vi "Experiment header-Save_Load config file data.vi"(5 "Header file actions":T1=enum."Write All", 7 "Header file sections":T22=enum."LOGIN", 8 "error in (no error)":errorcluster, 9 "All header parameters in":T2 {"VOLUME IMAGING"."Plane Mode" items=["XY Plane", "XZ Plane", "YZ Plane", "arbitraryplane"]; "VOLUME IMAGING"."Basic Image meta data"."Frame Size" items=["100X100"=100, "128X128"=128, "200X200"=200, "256X256"=256, "512X512"=512, "1024x1024"=1024, "2048x2048"=2048]; "AOL Z-STACK"."Hdr Basic Image meta data"."Frame Size" items=["100X100"=100, "128X128"=128, "200X200"=200, "256X256"=256, "512X512"=512, "1024x1024"=1024, "2048x2048"=2048]; "MOTOR Z-STACK"."Hdr Basic Image meta data"."Frame Size" items=["100X100"=100, "128X128"=128, "200X200"=200, "256X256"=256, "512X512"=512, "1024x1024"=1024, "2048x2048"=2048]; "FUNCTIONAL IMAGING"."Plane Mode" items=["XY Plane", "XZ Plane", "YZ Plane", "arbitraryplane"]; "FUNCTIONAL IMAGING"."Basic Image meta data"."Frame Size" items=["100X100"=100, "128X128"=128, "200X200"=200, "256X256"=256, "512X512"=512, "1024x1024"=1024, "2048x2048"=2048]; "TIME SERIES"."Basic Image meta data"."Frame Size" items=["100X100"=100, "128X128"=128, "200X200"=200, "256X256"=256, "512X512"=512, "1024x1024"=1024, "2048x2048"=2048]}, 11 "Experiment data folder path":path) -> (0 "error out":errorcluster, 1 "All header parameters out":T2 {"VOLUME IMAGING"."Plane Mode" items=["XY Plane", "XZ Plane", "YZ Plane", "arbitraryplane"]; "VOLUME IMAGING"."Basic Image meta data"."Frame Size" items=["100X100"=100, "128X128"=128, "200X200"=200, "256X256"=256, "512X512"=512, "1024x1024"=1024, "2048x2048"=2048]; "AOL Z-STACK"."Hdr Basic Image meta data"."Frame Size" items=["100X100"=100, "128X128"=128, "200X200"=200, "256X256"=256, "512X512"=512, "1024x1024"=1024, "2048x2048"=2048]; "MOTOR Z-STACK"."Hdr Basic Image meta data"."Frame Size" items=["100X100"=100, "128X128"=128, "200X200"=200, "256X256"=256, "512X512"=512, "1024x1024"=1024, "2048x2048"=2048]; "FUNCTIONAL IMAGING"."Plane Mode" items=["XY Plane", "XZ Plane", "YZ Plane", "arbitraryplane"]; "FUNCTIONAL IMAGING"."Basic Image meta data"."Frame Size" items=["100X100"=100, "128X128"=128, "200X200"=200, "256X256"=256, "512X512"=512, "1024x1024"=1024, "2048x2048"=2048]; "TIME SERIES"."Basic Image meta data"."Frame Size" items=["100X100"=100, "128X128"=128, "200X200"=200, "256X256"=256, "512X512"=512, "1024x1024"=1024, "2048x2048"=2048]})   [LabVIEW 2020]
doc: "This self-contained module handles all header files save/write operations.\nIt can generate a number of different header files containing different parameters.\nEach different type of header file has its own type defined cluster of parameters.\nThe functionality is fully self-scalable such as when new parameters are added or parameters are deleted or renamed in the typedef clusters this is all handled automatically without the need for further updates to this module."
uses:
  <vilib>/Utility/config.llb/NI_LVConfig.lvlib
  <vilib>/Utility/config.llb/Write Key (Double).vi
  Typedefs/Header file type enum.ctl
  Typedefs/Header subclusters/Header params -Login.ctl
  Misc/Experiment Type.ctl
  Typedefs/Header subclusters/Header params-Global Parameters.ctl
  Typedefs/Header subclusters/Header params-Imaging Modes.ctl
  Typedefs/Header subclusters/Header params-Basic image meta data.ctl
  Typedefs/Header subclusters/Header params-Time Series.ctl
  Typedefs/Header subclusters/Header params-Functional Imaging.ctl
  Typedefs/Reference source.ctl
  Typedefs/Header subclusters/Header params-Movement correction.ctl
  Typedefs/Header subclusters/Header params-Calibration Setup.ctl
  Typedefs/Header subclusters/Header params-statistics.ctl
  Misc/Biology Information.ctl
  Typedefs/Header subclusters/Header params-Motor Z-stack.ctl
  Typedefs/Header subclusters/Header params-AOL Z-stack.ctl
  Typedefs/Header parameters cluster-ALL.ctl
  Typedefs/Header file actions.ctl
  <vilib>/Utility/config.llb/Read Key (Double).vi
  Typedefs/Functional Mode.ctl
  Typedefs/AOL modes.ctl
  Typedefs/Plane Mode.ctl
  Typedefs/Frame Size.ctl
  Typedefs/Header subclusters/Header params-calibration data.ctl
  Typedefs/Header file sections.ctl
panel:
  out "error":errorcluster
  # "Actual FOV ------>\n(not norm FOFV)"
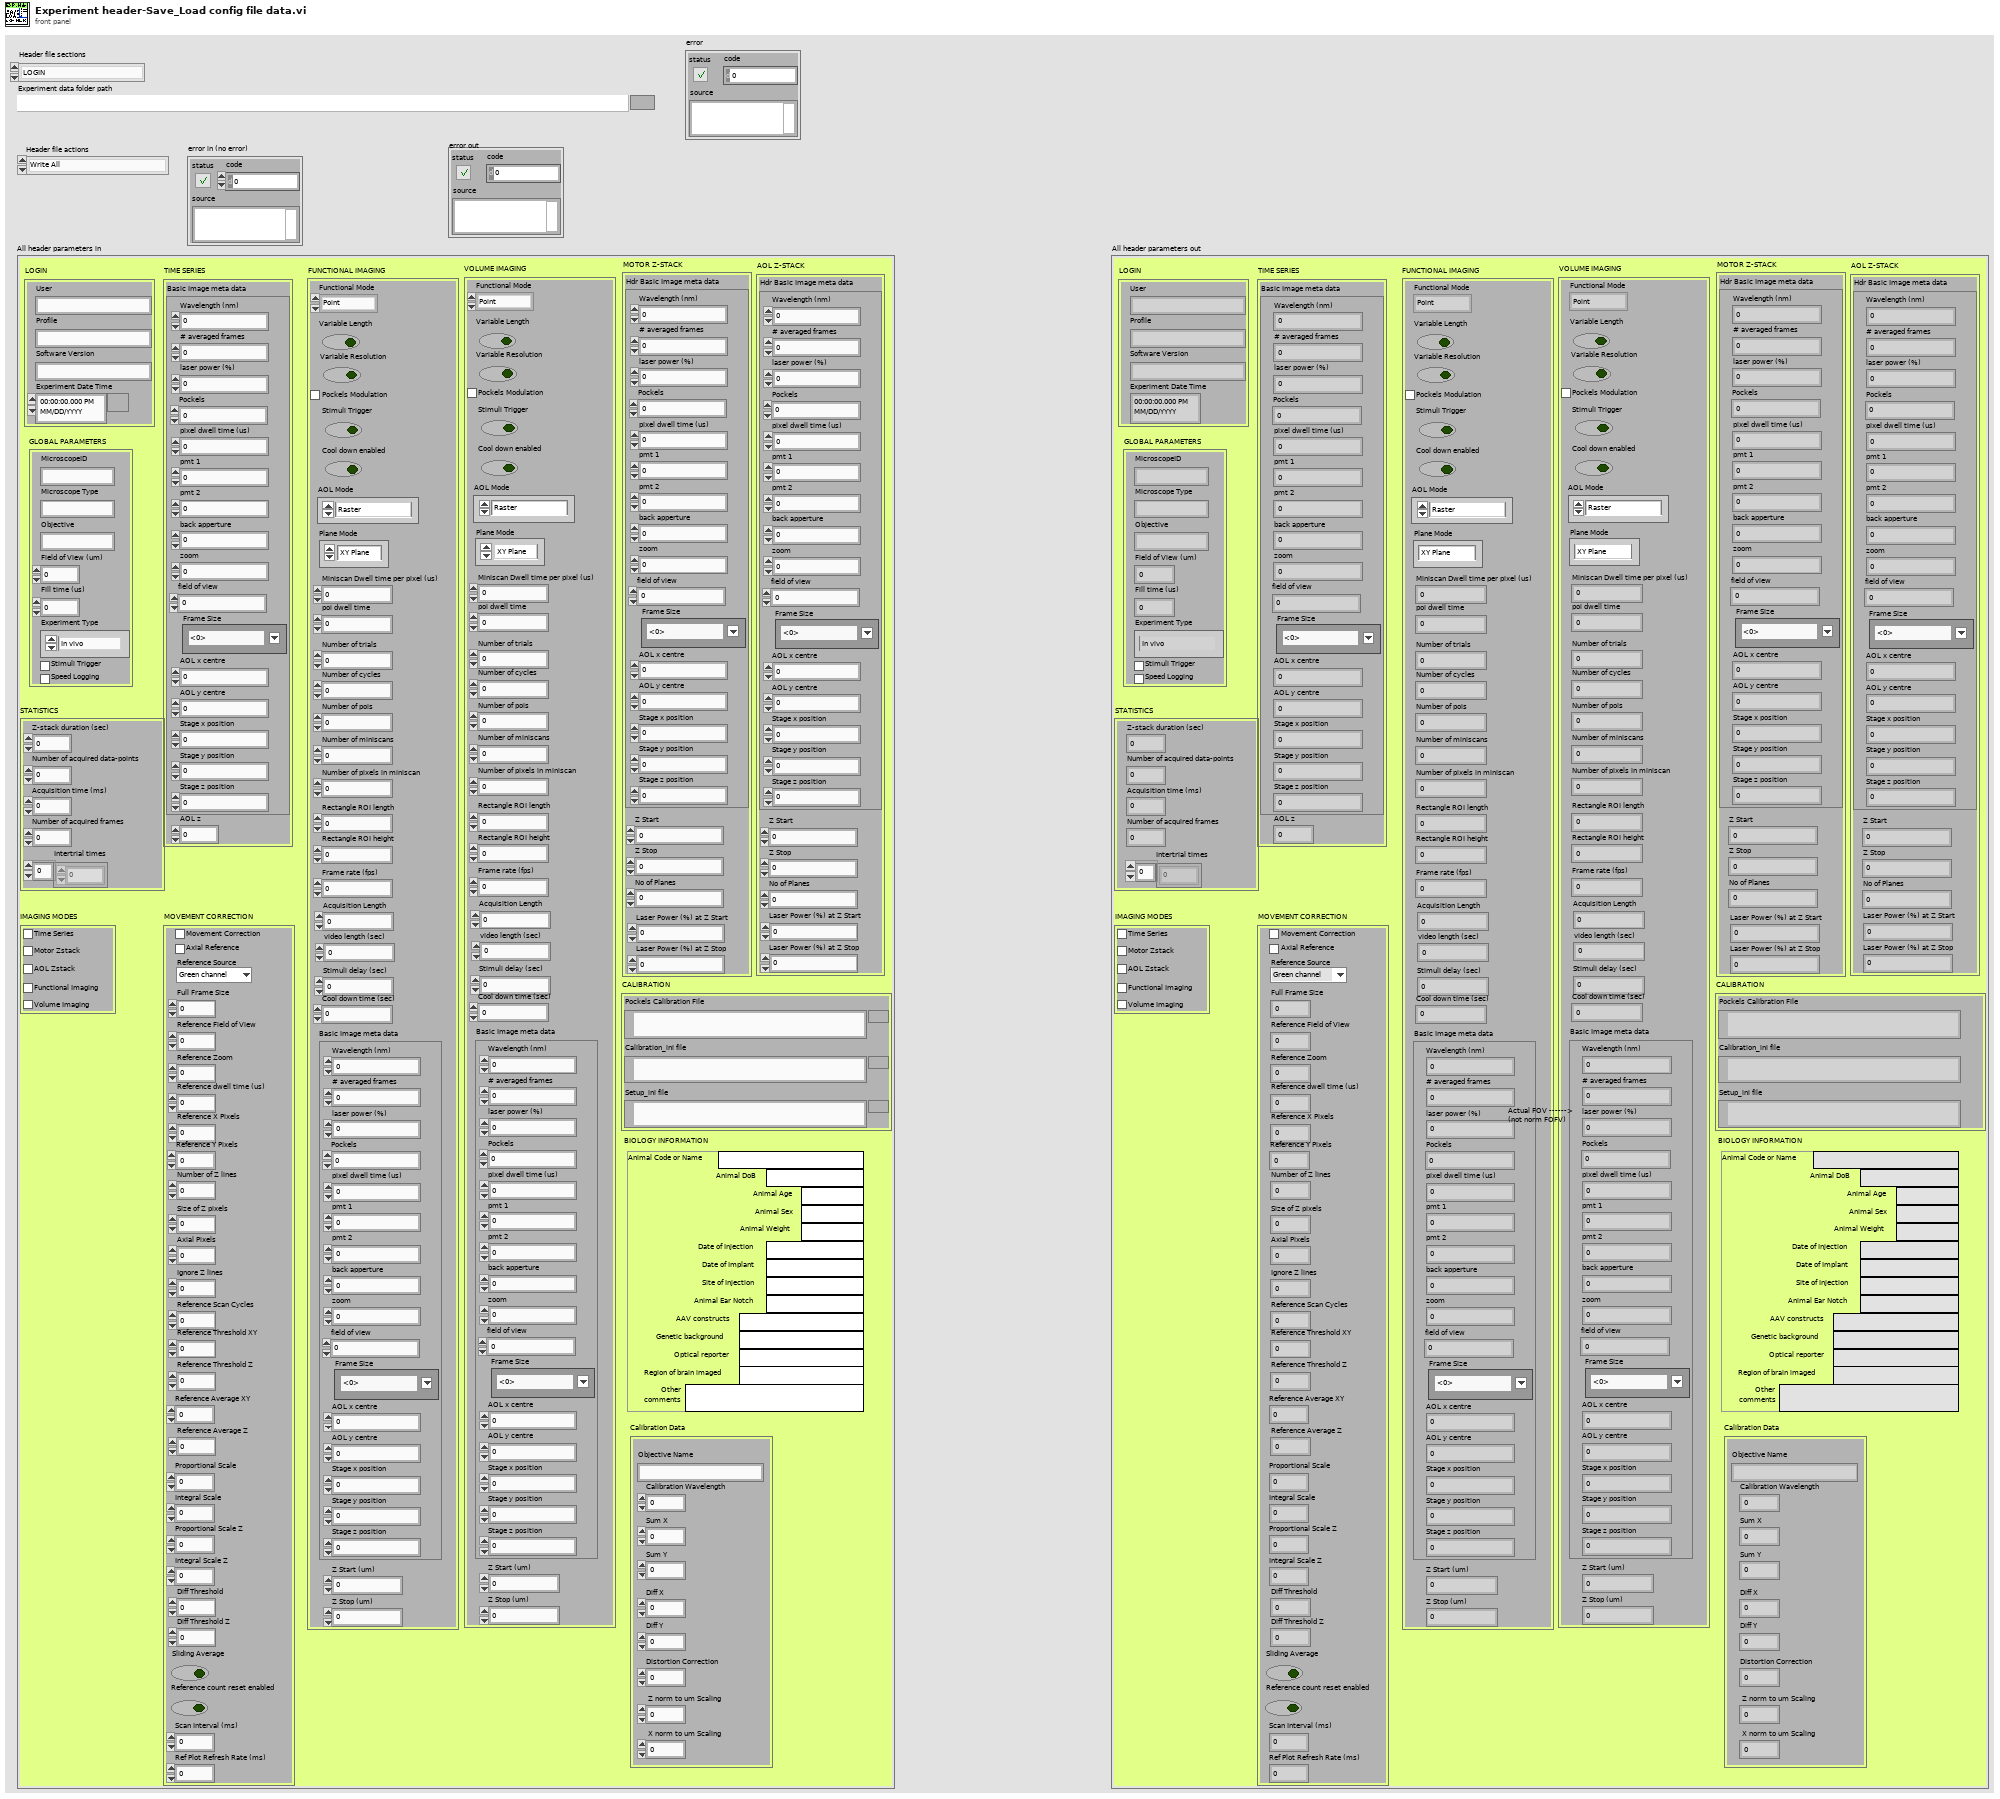
[diagram p1: front panel]
types:
  T1 = typedef "Header file actions.ctl" = enum16{"Create", "Open", "Read All", "Read Section", "Write All", "Write Section", "Close"}
  T2 = typedef "Header parameters cluster-ALL.ctl" = cluster{"LOGIN":T3, "GLOBAL PARAMETERS":T4, "IMAGING MODES":T6, "TIME SERIES":T7, "MOTOR Z-STACK ":T10, "AOL Z-STACK":T11, "FUNCTIONAL IMAGING":T12, "VOLUME IMAGING":T12, "MOVEMENT CORRECTION":T16, "CALIBRATION":T18, "STATISTICS":T19, "BIOLOGY INFORMATION":T20, "Calibration Data":T21}
  T3 = typedef "Header params -Login.ctl" = cluster{"User":string, "Profile":string, "Software Version":string, "Experiment Date Time":timestamp}
  T4 = typedef "Header params-Global Parameters.ctl" = cluster{"MicroscopeID":string, "Microscope Type":string, "Objective":string, "Field of View (um)":dbl, "Fill time (us)":dbl, "Experiment Type":T5, "Stimuli Trigger":bool, "Speed Logging":bool}
  T5 = typedef "Experiment Type.ctl" = enum16{"In vivo", "In vitro", "Testing", "Calibration", "Other"}
  T6 = typedef "Header params-Imaging Modes.ctl" = cluster{"Time Series":bool, "Motor Zstack":bool, "AOL Zstack":bool, "Functional Imaging":bool, "Volume Imaging":bool}
  T7 = typedef "Header params-Time Series.ctl" = cluster{"Basic Image meta data":T8, "AOL z":dbl}
  T8 = typedef "Header params-Basic image meta data.ctl" = cluster{"Wavelength (nm)":dbl, "# averaged frames":dbl, "laser power (%)":dbl, "Pockels":dbl, "pixel dwell time (us)":dbl, "pmt 1":dbl, "pmt 2":dbl, "back apperture":dbl, "zoom":dbl, "field of view":dbl, "Frame Size":T9, "AOL x centre":dbl, "AOL y centre":dbl, "Stage x position":dbl, "Stage y position":dbl, "Stage z position":dbl}
  T9 = typedef "Frame Size.ctl" = u16
  T10 = typedef "Header params-Motor Z-stack.ctl" = cluster{"Hdr Basic Image meta data":T8, "Z Start":dbl, "Z Stop":dbl, "No of Planes":i32, "Laser Power (%) at Z Start":dbl, "Laser Power (%) at Z Stop":dbl}
  T11 = typedef "Header params-AOL Z-stack.ctl" = cluster{"Hdr Basic Image meta data":T8, "Z Start":dbl, "Z Stop":dbl, "No of Planes":i32, "Laser Power (%) at Z Start":dbl, "Laser Power (%) at Z Stop":dbl}
  T12 = typedef "Header params-Functional Imaging.ctl" = cluster{"Functional Mode":T13, "Variable Length":bool, "Variable Resolution":bool, "Pockels Modulation":bool, "Stimuli Trigger":bool, "Cool down enabled":bool, "AOL Mode":T14, "Plane Mode":T15, "Miniscan Dwell time per pixel (us)":dbl, "poi dwell time":dbl, "Number of trials":dbl, "Number of cycles":dbl, "Number of pois":dbl, "Number of miniscans":dbl, "Number of pixels in miniscan":dbl, "Rectangle ROI length":dbl, "Rectangle ROI height":dbl, "Frame rate (fps)":dbl, "Acquisition Length":dbl, "video length (sec)":dbl, "Stimuli delay (sec)":dbl, "Cool down time (sec)":dbl, "Basic Image meta data":T8, "Z Start (um)":dbl, "Z Stop (um)":dbl}
  T13 = typedef "Functional Mode.ctl" = enum16{"Point", "Line", "Patch", "Plane", "Volume"}
  T14 = typedef "AOL modes.ctl" = enum16{"Raster", "Structural", "Pointing", "Mini Scan", "Alignment"}
  T15 = typedef "Plane Mode.ctl" = u16
  T16 = typedef "Header params-Movement correction.ctl" = cluster{"Movement Correction":bool, "Axial Reference":bool, "Reference Source":T17, "Full Frame Size":dbl, "Reference Field of View":dbl, "Reference Zoom":dbl, "Reference dwell time (us)":dbl, "Reference X Pixels":dbl, "Reference Y Pixels":dbl, "Number of Z lines":dbl, "Size of Z pixels":dbl, "Axial Pixels":dbl, "Ignore Z lines":dbl, "Reference Scan Cycles":dbl, "Reference Threshold XY":dbl, "Reference Threshold Z":dbl, "Reference Average XY":dbl, "Reference Average Z":dbl, "Proportional Scale":dbl, "Integral Scale":dbl, "Proportional Scale Z":dbl, "Integral Scale Z":dbl, "Diff Threshold":dbl, "Diff Threshold Z":dbl, "Sliding Average":bool, "Reference count reset enabled":bool, "Scan Interval (ms)":dbl, "Ref Plot Refresh Rate (ms)":dbl}
  T17 = typedef "Reference source.ctl" = enum16{"Green channel", "Red channel"}
  T18 = typedef "Header params-Calibration Setup.ctl" = cluster{"Pockels Calibration File":path, "Calibration_ini file":path, "Setup_ini file":path}
  T19 = typedef "Header params-statistics.ctl" = cluster{"Z-stack duration (sec)":dbl, "Number of acquired data-points":dbl, "Acquisition time (ms)":dbl, "Number of acquired frames":dbl, "Intertrial times":dbl[]}
  T20 = typedef "Biology Information.ctl" = cluster{"Animal Code or Name":string, "Animal DoB":string, "Animal Age":string, "Animal Sex":string, "Animal Weight":string, "Date of Injection":string, "Date of Implant":string, "Site of Injection":string, "Animal Ear Notch":string, "AAV constructs":string, "Genetic background":string, "Optical reporter":string, "Region of brain imaged":string, "Other \ncomments":string}
  T21 = typedef "Header params-calibration data.ctl" = cluster{"Objective Name":string, "Calibration Wavelength":dbl, "Sum X":dbl, "Sum Y":dbl, "Diff X":dbl, "Diff Y":dbl, "Distortion Correction":dbl, " Z norm to um Scaling":dbl, " X norm to um Scaling":dbl}
  T22 = typedef "Header file sections.ctl" = enum16{"ALL SECTIONS", "LOGIN", "GLOBAL PARAMETERS", "CALIBRATION DATA", "IMAGING MODES", "TIME SERIES", "MOTOR Z-STACK", "AOL Z-STACK", "FUNCTIONAL IMAGING", "VOLUME IMAGING", "ARBOREAL SCANNING", "MULTIBEAM PARAMETERS", "MOVEMENT CORRECTION", "CALIBRATION", "STATISTICS", "BIOLOGY INFORMATION", "PARAMETER SWEEP"}
  T23 = typedef "Header file section refs.ctl" = cluster{"Section Name":string, "Section Ref":refnum<vi>, "Section Controls[]":refnum<vi>[]}
  T24 = typedef "Fixed strings.ctl" = cluster{"ROI file name":string, "Normalised ROI file name":string, "Zplane Pockels values file name":string, "Functional data folder name":string, "Experiment Header file name":string, "Z-stack images folder name":string, "Groups setup rel. path":string, "Groups text file rel. path":string, "TDMS files folder name (F.img)":string, "TDMS files folder name (V.acq)":string, "TDMS files folder name (Pl.acq)":string, "Cycle rel times sequence file":string, "Dynamically called VIs folder name":string, "Time Series folder base name":string, "Parameter Sweep":string}
  T25 = typedef "Header parameters cluster-ALL.ctl" = cluster{"LOGIN":T3, "GLOBAL PARAMETERS":T4, "IMAGING MODES":T6, "TIME SERIES":T7, "MOTOR Z-STACK ":T10, "AOL Z-STACK":T11, "FUNCTIONAL IMAGING":T12, "VOLUME IMAGING":T12, "MOVEMENT CORRECTION":T16, "CALIBRATION":T18, "STATISTICS":T19, "BIOLOGY INFORMATION":T20, "Calibration Data":T21, "Parameter Sweep Settings":T26}
  T26 = typedef "Header params-Parameter Sweep.ctl" = cluster{"Parameter Sweep Steps":T27, "Parameter Sweep":T28, "# Sw. Planes":i32, "Basic image meta-data":T8}
  T27 = typedef "Parameter Sweep Steps.ctl" = cluster{"MB Sep Start":dbl, "MB Sep Stop":dbl, "MB Sep Step":dbl}
  T28 = typedef "Parameter sweep modes.ctl" = enum16{"None Selected", "Dwell Time [us]"}
  T29 = typedef "Header file type enum.ctl" = enum16{"All parameters", "Login", "Global Parameters", "Imaging Modes", "Time Series", "Motor Zstack", "AOL Zstack", "Functional Imaging", "Movement Correction", "Calibration Setup", "Statistics", "Biology Information"}
  T30 = typedef "NI_LVConfig.lvlib/Config Data RefNum.ctl" = refnum<k1>
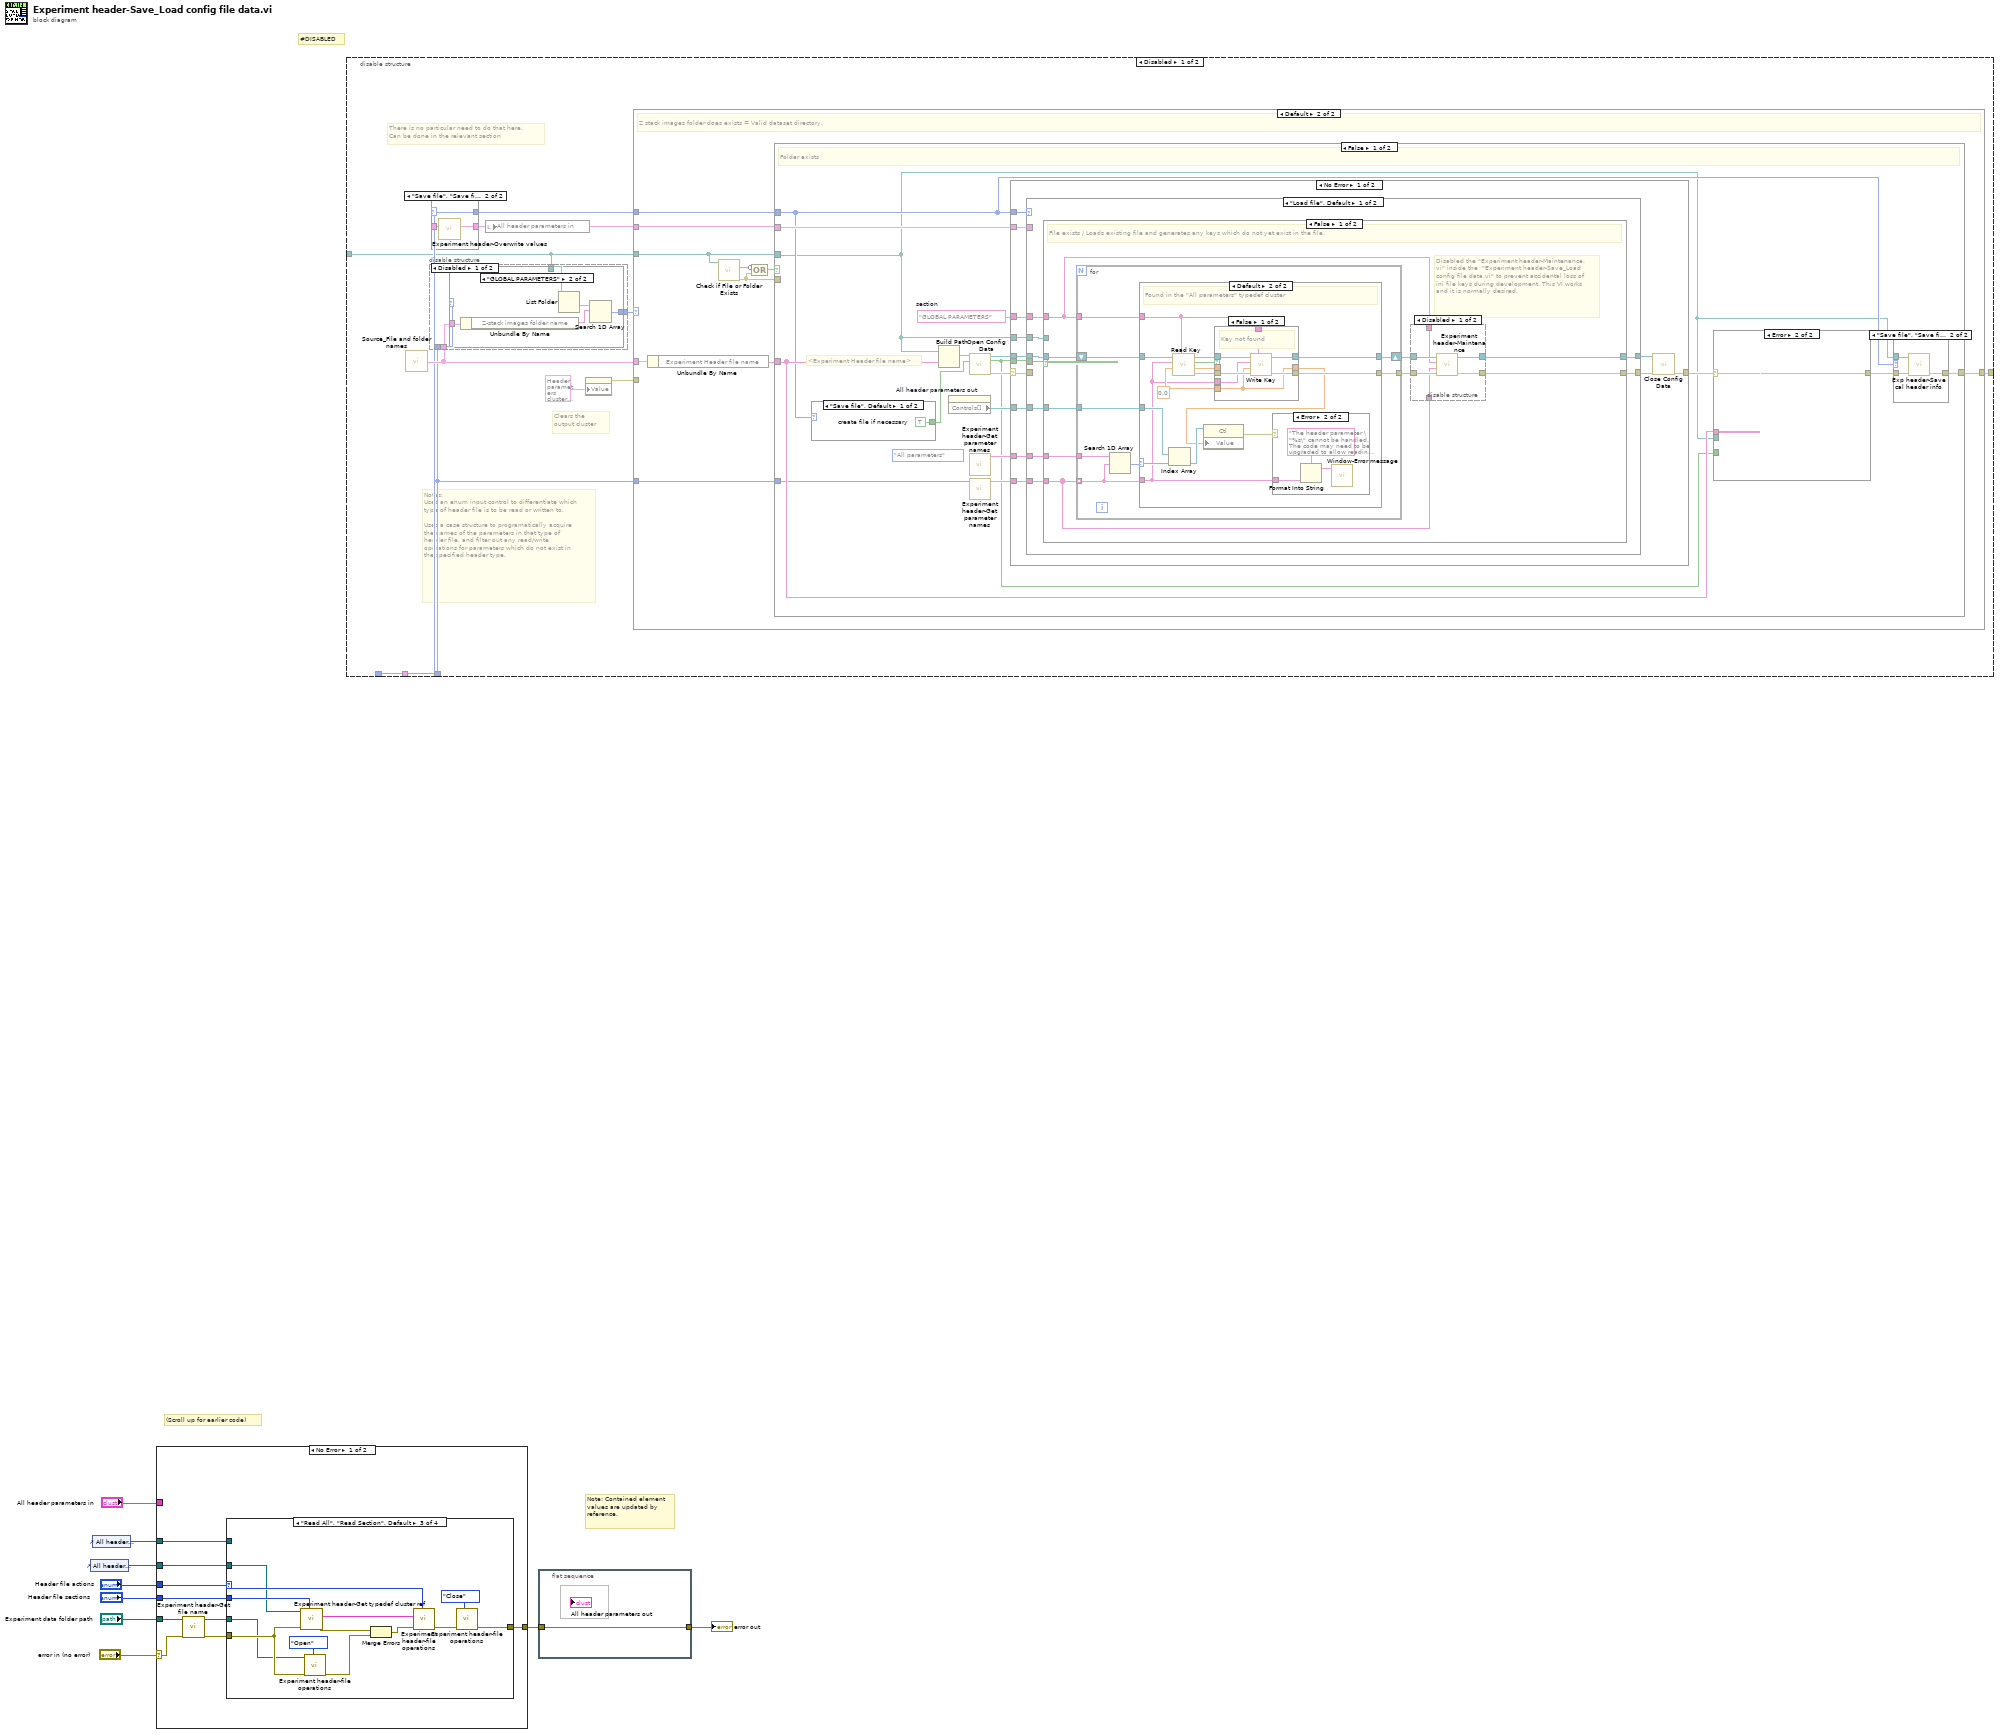
[diagram p0: block diagram]
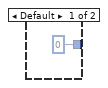
[diagram p3: hidden frame]
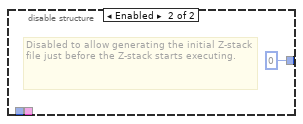
[diagram p4: hidden frame]
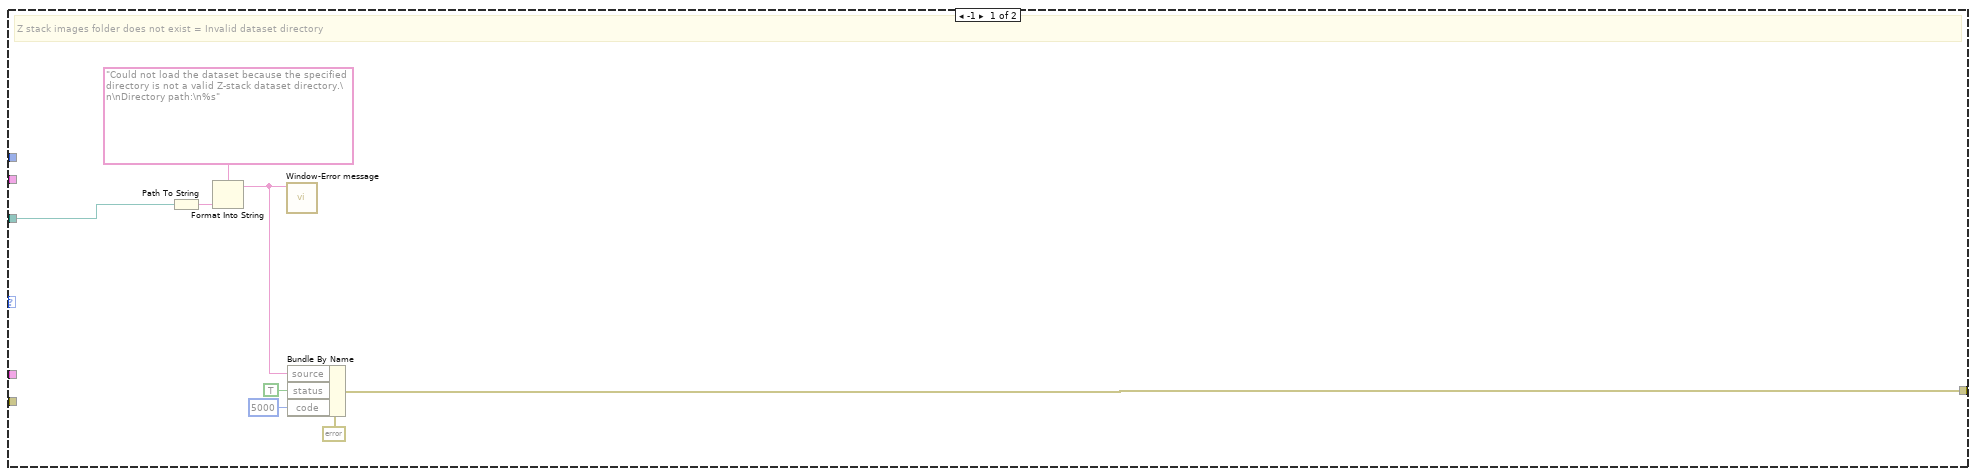
[diagram p5: hidden frame]
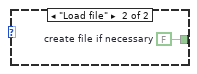
[diagram p7: hidden frame]
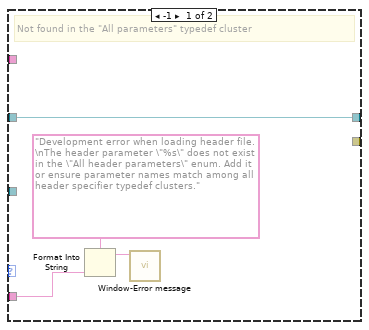
[diagram p9: hidden frame]
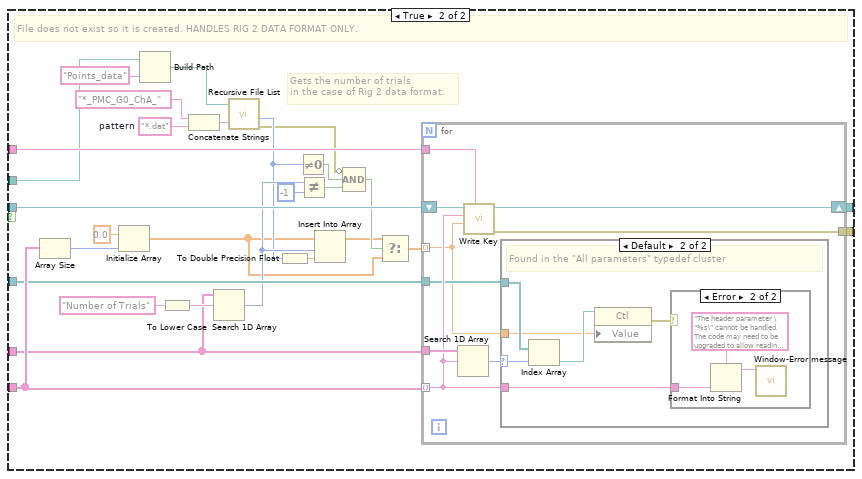
[diagram p12: hidden frame]
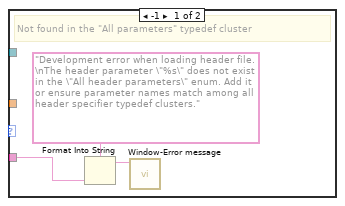
[diagram p13: hidden frame]
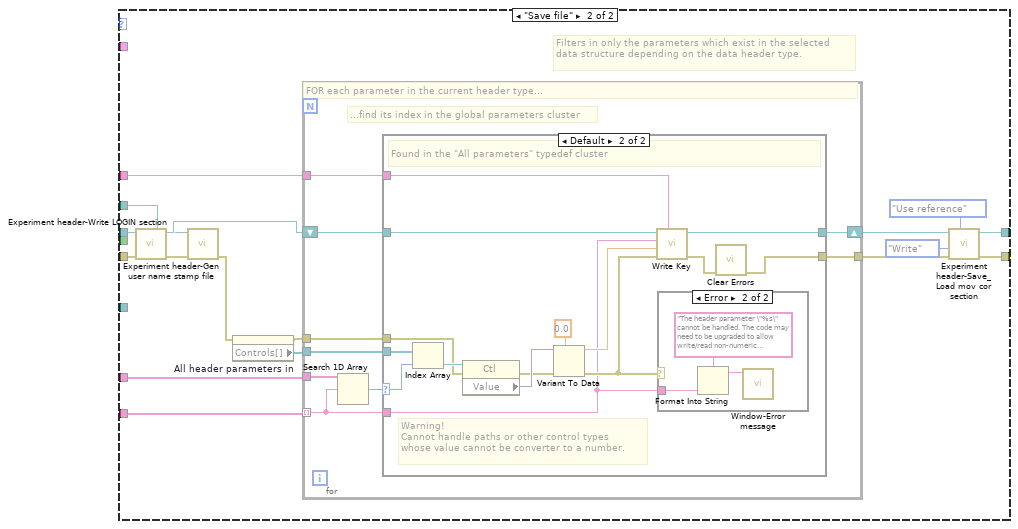
[diagram p15: hidden frame]
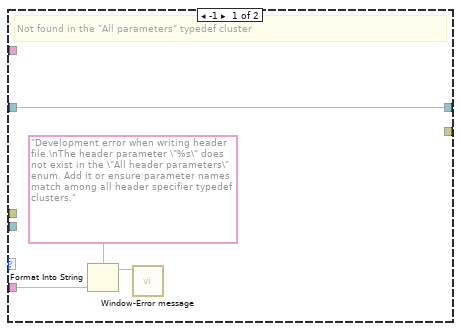
[diagram p16: hidden frame]
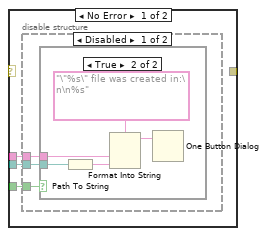
[diagram p19: hidden frame]
diagram:
  # "Note: Contained element values are updated by reference."
  # "(Scroll up for earlier code)"
  # "#DISABLED"
  n1 = control-ref of="All header parameters out"() -> (w3:refnum<vi>)
  n2 = control-ref of="All header parameters in"() -> (w4:refnum<vi>)
  n3 = case shown="No Error" "error in (no error)" {
    selector: "error in (no error)" -> [w11 w53]
    tunnel: [w10 w53] -> w2
    tunnel: "Header file sections" -> [w15 _]
    tunnel: "All header parameters in" -> [_ _]
    tunnel: "Experiment data folder path" -> [w18 _]
    tunnel: "Header file actions" -> [w14 _]
    tunnel: w4 -> [w13 _]
    tunnel: w3 -> [w12 _]
    frame No Error {
      n4 = call "Experiment header-Get file name.vi"("error in (no error)"=w11, "Experiment data folder path"=w18) -> ("error out"=w17:errorcluster, "Header File Path"=w16:path)  [unwired: 8 in]
      n5 = case shown="\"Read All\", \"Read Section\", Default" w14 {
        selector: w14 -> [w21 w34 w48 _]
        tunnel: w17 -> [w22 w27 w45 w52]
        tunnel: w16 -> [w20 w33 w38 _]
        tunnel: w15 -> [_ w35 w47 _]
        tunnel: w13 -> [_ w23 _ _]
        tunnel: w12 -> [_ _ w37 _]
        tunnel: [w19 w24 w40 w50] -> w10
        frame "Create" {
          n6 = call "Experiment header-file operations.vi"("Header file actions"=w21, "error in (no error)"=w22, "Path"=w20) -> ("error out"=w19:errorcluster)  [unwired: 8 in]
        }
        frame "Write All", "Write Section" {
          n7 = call "Experiment header-Gen user name stamp file.vi"("error in (no error)"=w27, "Experiment data folder path"=w33) -> ("error out"=→"error":errorcluster)  [unwired: 9 in]
          n8 = call "Experiment header-Get typedef cluster ref.vi"("Header file sections"=w35, "All header parameters / Header module interface cluster"=w23) -> ("error out"=w31:errorcluster, "Section Refs"=w36:T23[])  [unwired: 6 in, 2 out]
          n9 = call "Experiment header-file operations.vi"("Header file actions"=Header_file_actions."Open", "error in (no error)"=w27, "Path"=w33) -> ("error out"=w30:errorcluster)  [unwired: 8 in]
          n10 = Merge Errors(w31, w30) -> (w29:errorcluster)
          n11 = call "Experiment header-file operations.vi"("Header file actions"=w34, "error in (no error)"=w29, "Section Refs"=w36) -> ("error out"=w25:errorcluster)  [unwired: 8 in]
          n12 = call "Experiment header-file operations.vi"("Header file actions"=Header_file_actions."Close", "error in (no error)"=w25) -> ("error out"=w24:errorcluster)  [unwired: 9 in]
        }
        frame "Read All", "Read Section", Default {
          n13 = call "Experiment header-Get typedef cluster ref.vi"("Header file sections"=w47, "error in (no error)"=w45, "All header parameters / Header module interface cluster"=w37) -> ("error out"=w44:errorcluster, "Section Refs"=w49:T23[])  [unwired: 5 in, 2 out]
          n14 = call "Experiment header-file operations.vi"("Header file actions"=Header_file_actions."Open", "error in (no error)"=w45, "Path"=w38) -> ("error out"=w42:errorcluster)  [unwired: 8 in]
          n15 = Merge Errors(w44, w42) -> (w43:errorcluster)
          n16 = call "Experiment header-file operations.vi"("Header file actions"=w48, "error in (no error)"=w43, "Section Refs"=w49) -> ("error out"=w39:errorcluster)  [unwired: 8 in]
          n17 = call "Experiment header-file operations.vi"("Header file actions"=Header_file_actions."Close", "error in (no error)"=w39) -> ("error out"=w40:errorcluster)  [unwired: 9 in]
        }
        frame "Close" {
          n18 = call "Experiment header-file operations.vi"("Header file actions"=Header_file_actions."Close", "error in (no error)"=w52) -> ("error out"=w50:errorcluster)  [unwired: 9 in]
        }
      }
    }
    frame Error {
    }
  }
  n19 = disable-structure shown="Disabled" {
    disable-tunnel: [w64 _] -> _
    disable-tunnel: _ -> [w59 _]
    disable-tunnel: _ -> [w58 _]
    disable-tunnel: _ -> [w57 _]
    disable-tunnel: _ -> [w54 _]
    frame Disabled {
      # "There is no particular need to do that here.\nCan be done in the relevant section"
      # "Clears the output cluster"
      # "Notes:\nUses an enum input control to differentiate which type of header file is to be read or written to.\n\nUses a case structure to programatically acquire the names of the parameters in that type of header file, and filter out any read/write operations for parameters which do not exist in the specified header type."
      n20 = call "Source_File and folder names.vi"() -> ("Fixed strings"=w62:T24)  [unwired: 1 in]
      n21 = disable-structure shown="Disabled" {
        disable-tunnel: w57 -> [w73 _]
        disable-tunnel: [w72 0 ("index of element")] -> w63
        disable-tunnel: w62 -> [w71 _]
        disable-tunnel: w54 -> [w70 _]
        frame Disabled {
          n22 = case shown="\"GLOBAL PARAMETERS\"" w70 {
            tunnel: w73 -> [_ w78]
            tunnel: [0 ("index of element") w77] -> w72
            tunnel: w71 -> [_ w75]
            frame Default {
            }
            frame "GLOBAL PARAMETERS" {
              n23 = Unbundle By Name(w75) -> ("Z-stack images folder name"=w76:string)
              n24 = List Folder(path=w78) -> (folder names=w79:string[])  [unwired: 3 in, 3 out]
              n25 = Search 1D Array(1D array=w79, element=w76) -> (index of element=w77:i32)  [unwired: 1 in]
            }
          }
        }
        frame Enabled {
          # "Disabled to allow generating the initial Z-stack file just before the Z-stack starts executing."
        }
      }
      n26 = case shown="\"Save file\", \"Save file as\"" w59 {
        selector: w59 -> [w66 w68]
        tunnel: [w65 w69] -> w56
        tunnel: [w66 w68] -> w60
        tunnel: w58 -> [w65 w67]
        frame Default {
        }
        frame "Save file", "Save file as" {
          n27 = call "Experiment header-Overwrite values.vi"("All header parameters in"=w67) -> ("All header parameters (FOV converted to um)"=w69:T25)  [unwired: 9 in, 1 out]
        }
      }
      n28 = local write "All header parameters in"(w56) -> ()
      n29 = property on="All header parameters out" class="Clust (strict)"("Value"=T2 {"LOGIN"={"User"="", "Profile"="", "Software Version"="", "Experiment Date Time"=timestamp(0 s since 1904-01-01)}, "GLOBAL PARAMETERS"={"MicroscopeID"="", "Microscope Type"="", "Objective"="", "Field of View (um)"=0.0, "Fill time (us)"=0.0, "Experiment Type"=enum."In vivo", "Stimuli Trigger"=FALSE, "Speed Logging"=FALSE}, "IMAGING MODES"={"Time Series"=FALSE, "Motor Zstack"=FALSE, "AOL Zstack"=FALSE, "Functional Imaging"=FALSE, "Volume Imaging"=FALSE}, "TIME SERIES"={"Basic Image meta data"={"Wavelength (nm)"=0.0, "# averaged frames"=0.0, "laser power (%)"=0.0, "Pockels"=0.0, "pixel dwell time (us)"=0.0, "pmt 1"=0.0, "pmt 2"=0.0, "back apperture"=0.0, "zoom"=0.0, "field of view"=0.0, "Frame Size"=0, "AOL x centre"=0.0, "AOL y centre"=0.0, "Stage x position"=0.0, "Stage y position"=0.0, "Stage z position"=0.0}, "AOL z"=0.0}, "MOTOR Z-STACK "={"Hdr Basic Image meta data"={"Wavelength (nm)"=0.0, "# averaged frames"=0.0, "laser power (%)"=0.0, "Pockels"=0.0, "pixel dwell time (us)"=0.0, "pmt 1"=0.0, "pmt 2"=0.0, "back apperture"=0.0, "zoom"=0.0, "field of view"=0.0, "Frame Size"=0, "AOL x centre"=0.0, "AOL y centre"=0.0, "Stage x position"=0.0, "Stage y position"=0.0, "Stage z position"=0.0}, "Z Start"=0.0, "Z Stop"=0.0, "No of Planes"=0, "Laser Power (%) at Z Start"=0.0, "Laser Power (%) at Z Stop"=0.0}, "AOL Z-STACK"={"Hdr Basic Image meta data"={"Wavelength (nm)"=0.0, "# averaged frames"=0.0, "laser power (%)"=0.0, "Pockels"=0.0, "pixel dwell time (us)"=0.0, "pmt 1"=0.0, "pmt 2"=0.0, "back apperture"=0.0, "zoom"=0.0, "field of view"=0.0, "Frame Size"=0, "AOL x centre"=0.0, "AOL y centre"=0.0, "Stage x position"=0.0, "Stage y position"=0.0, "Stage z position"=0.0}, "Z Start"=0.0, "Z Stop"=0.0, "No of Planes"=0, "Laser Power (%) at Z Start"=0.0, "Laser Power (%) at Z Stop"=0.0}, "FUNCTIONAL IMAGING"={"Functional Mode"=enum."Point", "Variable Length"=FALSE, "Variable Resolution"=FALSE, "Pockels Modulation"=FALSE, "Stimuli Trigger"=FALSE, "Cool down enabled"=FALSE, "AOL Mode"=enum."Raster", "Plane Mode"=0, "Miniscan Dwell time per pixel (us)"=0.0, "poi dwell time"=0.0, "Number of trials"=0.0, "Number of cycles"=0.0, "Number of pois"=0.0, "Number of miniscans"=0.0, "Number of pixels in miniscan"=0.0, "Rectangle ROI length"=0.0, "Rectangle ROI height"=0.0, "Frame rate (fps)"=0.0, "Acquisition Length"=0.0, "video length (sec)"=0.0, "Stimuli delay (sec)"=0.0, "Cool down time (sec)"=0.0, "Basic Image meta data"={"Wavelength (nm)"=0.0, "# averaged frames"=0.0, "laser power (%)"=0.0, "Pockels"=0.0, "pixel dwell time (us)"=0.0, "pmt 1"=0.0, "pmt 2"=0.0, "back apperture"=0.0, "zoom"=0.0, "field of view"=0.0, "Frame Size"=0, "AOL x centre"=0.0, "AOL y centre"=0.0, "Stage x position"=0.0, "Stage y position"=0.0, "Stage z position"=0.0}, "Z Start (um)"=0.0, "Z Stop (um)"=0.0}, "VOLUME IMAGING"={"Functional Mode"=enum."Point", "Variable Length"=FALSE, "Variable Resolution"=FALSE, "Pockels Modulation"=FALSE, "Stimuli Trigger"=FALSE, "Cool down enabled"=FALSE, "AOL Mode"=enum."Raster", "Plane Mode"=0, "Miniscan Dwell time per pixel (us)"=0.0, "poi dwell time"=0.0, "Number of trials"=0.0, "Number of cycles"=0.0, "Number of pois"=0.0, "Number of miniscans"=0.0, "Number of pixels in miniscan"=0.0, "Rectangle ROI length"=0.0, "Rectangle ROI height"=0.0, "Frame rate (fps)"=0.0, "Acquisition Length"=0.0, "video length (sec)"=0.0, "Stimuli delay (sec)"=0.0, "Cool down time (sec)"=0.0, "Basic Image meta data"={"Wavelength (nm)"=0.0, "# averaged frames"=0.0, "laser power (%)"=0.0, "Pockels"=0.0, "pixel dwell time (us)"=0.0, "pmt 1"=0.0, "pmt 2"=0.0, "back apperture"=0.0, "zoom"=0.0, "field of view"=0.0, "Frame Size"=0, "AOL x centre"=0.0, "AOL y centre"=0.0, "Stage x position"=0.0, "Stage y position"=0.0, "Stage z position"=0.0}, "Z Start (um)"=0.0, "Z Stop (um)"=0.0}, "MOVEMENT CORRECTION"={"Movement Correction"=FALSE, "Axial Reference"=FALSE, "Reference Source"=enum."Green channel", "Full Frame Size"=0.0, "Reference Field of View"=0.0, "Reference Zoom"=0.0, "Reference dwell time (us)"=0.0, "Reference X Pixels"=0.0, "Reference Y Pixels"=0.0, "Number of Z lines"=0.0, "Size of Z pixels"=0.0, "Axial Pixels"=0.0, "Ignore Z lines"=0.0, "Reference Scan Cycles"=0.0, "Reference Threshold XY"=0.0, "Reference Threshold Z"=0.0, "Reference Average XY"=0.0, "Reference Average Z"=0.0, "Proportional Scale"=0.0, "Integral Scale"=0.0, "Proportional Scale Z"=0.0, "Integral Scale Z"=0.0, "Diff Threshold"=0.0, "Diff Threshold Z"=0.0, "Sliding Average"=FALSE, "Reference count reset enabled"=FALSE, "Scan Interval (ms)"=0.0, "Ref Plot Refresh Rate (ms)"=0.0}, "CALIBRATION"={"Pockels Calibration File"=path "", "Calibration_ini file"=path "", "Setup_ini file"=path ""}, "STATISTICS"={"Z-stack duration (sec)"=0.0, "Number of acquired data-points"=0.0, "Acquisition time (ms)"=0.0, "Number of acquired frames"=0.0, "Intertrial times"=[]}, "BIOLOGY INFORMATION"={"Animal Code or Name"="", "Animal DoB"="", "Animal Age"="", "Animal Sex"="", "Animal Weight"="", "Date of Injection"="", "Date of Implant"="", "Site of Injection"="", "Animal Ear Notch"="", "AAV constructs"="", "Genetic background"="", "Optical reporter"="", "Region of brain imaged"="", "Other \ncomments"=""}, "Calibration Data"={"Objective Name"="", "Calibration Wavelength"=0.0, "Sum X"=0.0, "Sum Y"=0.0, "Diff X"=0.0, "Diff Y"=0.0, "Distortion Correction"=0.0, " Z norm to um Scaling"=0.0, " X norm to um Scaling"=0.0}} ("All header parameters out")) -> (error out=w61:errorcluster)  [unwired: 2 in, 1 out]
      n30 = case shown="Default" w63 {
        tunnel: [w81 w98] -> w64
        tunnel: w60 -> [_ w94]
        tunnel: w56 -> [_ w93]
        tunnel: w57 -> [w86 w92]
        tunnel: w62 -> [_ w90]
        tunnel: w54 -> [_ w89]
        tunnel: w61 -> [_ _]
        frame -1 {
          # "Z stack images folder does not exist = Invalid dataset directory"
          n31 = Path To String(path=w86) -> (string=w88:string)
          n32 = Format Into String(format string="Could not load the dataset because the specified directory is not a valid Z-stack dataset directory.\n\nDirectory path:\n%s" ("message"), w88) -> (resulting string=w82:string)  [unwired: 2 in, 1 out]
          n33 = call "Window-Error message.vi"("Message"=w82) -> ()  [unwired: 10 in, 1 out]
          n34 = Bundle By Name(cluster=errorcluster {"status"=FALSE, "code"=0, "source"=""} ("error out"), "source"=w82, "status"=TRUE, "code"=5000) -> (w81:errorcluster)
        }
        frame Default {
          # "Z stack images folder does exists = Valid dataset directory."
          n35 = Unbundle By Name(w90) -> ("Experiment Header file name"=w91:string)
          n36 = call <vilib>:"Check if File or Folder Exists.vi"("path"=w92) -> ("error out"=w95:errorcluster, "file or folder exists?"=w97:bool)  [unwired: 8 in, 1 out]
          n37 = Compound Arithmetic op=OR(invert w97, w95) -> (w96:bool)
          n38 = case shown="False" w96 {
            tunnel: [w102 w312] -> w98
            tunnel: w91 -> [w110 _]
            tunnel: w92 -> [w99 w313]
            tunnel: w95 -> [_ w311]
            tunnel: w94 -> [w100 _]
            tunnel: w93 -> [w115 _]
            tunnel: w89 -> [w109 _]
            frame False {
              w104 = "GLOBAL PARAMETERS"  # section
              (unwired) Header_file_type_enum."All parameters" ("Header file type")
              # "<Experiment Header file name>"
              # "Folder exists"
              n39 = case shown="\"Save file\", Default" w100 {
                tunnel: [w120 w121] -> w103
                frame "Save file", Default {
                  w120 = TRUE  # create file if necessary
                }
                frame "Load file" {
                  w121 = FALSE  # create file if necessary
                }
              }
              n40 = Build Path(base path=w99, name or relative path=w110) -> (appended path=w114:path)
              n41 = property on="All header parameters out" class="Clust (strict)"() -> ("Controls[]"=w106:refnum<vi>[])  [unwired: 2 in, 2 out]
              n42 = call <vilib>:"Open Config Data.vi"("create file if necessary (T)"=w103, "configuration file path"=w114) -> ("error out"=w107:errorcluster, "file created?"=w105:bool, "refnum"=w113:T30)  [unwired: 7 in]
              n43 = call "Experiment header-Get parameter names.vi"() -> ("Section Names"=w108:string[])  [unwired: 9 in, 2 out]
              n44 = call "Experiment header-Get parameter names.vi"("Section Refs"=w109) -> ("Section Names"=w111:string[])  [unwired: 8 in, 2 out]
              n45 = case shown="No Error" w107 {
                selector: w107 -> [w122 w298]
                tunnel: w104 -> [w134 _]
                tunnel: w100 -> [w133 _]
                tunnel: w115 -> [w132 _]
                tunnel: w113 -> [w131 _]
                tunnel: [w128 w298] -> w112
                tunnel: w111 -> [w127 _]
                tunnel: w99 -> [w126 _]
                tunnel: w105 -> [w125 _]
                tunnel: w108 -> [w124 _]
                tunnel: w106 -> [w123 _]
                frame No Error {
                  n46 = case shown="\"Load file\", Default" w133 {
                    tunnel: [w138 w260] -> w129
                    tunnel: w134 -> [w143 w266]
                    tunnel: w132 -> [_ _]
                    tunnel: w127 -> [w142 w265]
                    tunnel: w125 -> [w140 _]
                    tunnel: w131 -> [w141 w264]
                    tunnel: [w139 w258] -> w130
                    tunnel: w126 -> [w137 w252]
                    tunnel: w124 -> [w136 w263]
                    tunnel: w123 -> [w135 _]
                    tunnel: w122 -> [_ w254]
                    frame "Load file", Default {
                      n47 = case shown="False" w140 {
                        tunnel: w141 -> [w152 w228]
                        tunnel: w143 -> [w145 w227]
                        tunnel: w142 -> [w146 w216]
                        tunnel: [w149 w226] -> w139
                        tunnel: [w148 w225] -> w138
                        tunnel: w137 -> [_ w215]
                        tunnel: w136 -> [w147 w212]
                        tunnel: w135 -> [w144 w211]
                        frame False {
                          # "Disabled the \"Experiment header-Maintenance.vi\" inside the  \"Experiment header-Save_Load config file data.vi\" to prevent accidental loss of ini file keys during development. This VI works and it is normally desired."
                          # "File exists / Loads existing file and generates any keys which do not yet exist in the file."
                          n48 = for {
                            shift-right: [w167] -> w151
                            shift-left: w152 -> [w168]
                            tunnel: w145 -> [w166]
                            tunnel: [w165] -> w150
                            tunnel: w146 -> [w163] mode=indexing
                            tunnel: w147 -> [w164]
                            tunnel: w144 -> [w161]
                            n49 = Search 1D Array(1D array=w164, element=w163) -> (index of element=w162:i32)  [unwired: 1 in]
                            n50 = case shown="Default" w162 {
                              selector: w162 -> [_ w177]
                              tunnel: w168 -> [w170 w187]
                              tunnel: [w170 w185] -> w167
                              tunnel: w166 -> [_ w183]
                              tunnel: [_ w181] -> w165
                              tunnel: w163 -> [w169 w173]
                              tunnel: w161 -> [_ w176]
                              frame -1 {
                                # "Not found in the \"All parameters\" typedef cluster"
                                n51 = Format Into String(format string="Development error when loading header file.\nThe header parameter \"%s\" does not exist in the \"All header parameters\" enum. Add it or ensure parameter names match among all header specifier typedef clusters.", w169) -> (resulting string=w171:string)  [unwired: 2 in, 1 out]
                                n52 = call "Window-Error message.vi"("Message"=w171) -> ()  [unwired: 10 in, 1 out]
                              }
                              frame Default {
                                w179 = 0.0 ("default value")
                                # "Found in the \"All parameters\" typedef cluster"
                                n53 = Index Array(array=w176, index=w177) -> (element=w178:refnum<vi>)
                                n54 = call-poly <vilib>:"Read Key.vi"("section"=w183, "default value"=w179, "key"=w173, "refnum"=w187) -> ("error out"=w182:errorcluster, "value"=w184:dbl, "found?"=w180:bool, "refnum out"=w186:T30)  [unwired: 4 in]
                                n55 = case shown="False" w180 {
                                tunnel: w186 -> [w197 w200]
                                tunnel: [w196 w200] -> w185
                                tunnel: w184 -> [_ w199]
                                tunnel: [w192 w199] -> w175
                                tunnel: w183 -> [w195 _]
                                tunnel: w179 -> [w192 _]
                                tunnel: w182 -> [w194 w198]
                                tunnel: [w193 w198] -> w181
                                tunnel: w173 -> [w191 _]
                                frame False {
                                # "Key not found"
                                n56 = call-poly <vilib>:"Write Key.vi"("section"=w195, "error in (no error)"=w194, "value"=w192, "key"=w191, "refnum"=w197) -> ("error out"=w193:errorcluster, "refnum out"=w196:T30)  [unwired: 4 in, 1 out]
                                }
                                frame True {
                                # "Key found"
                                }
                                }
                                n57 = property class="Ctl"(reference=w178, "Value"=w175) -> (error out=w174:errorcluster)  [unwired: 1 in, 1 out]
                                n58 = case shown="Error" w174 {
                                tunnel: w173 -> [_ w189]
                                frame No Error {
                                }
                                frame Error {
                                n59 = Format Into String(format string="The header parameter \"%s\" cannot be handled. The code may need to be upgraded to allow reading non-numeric parameter values from the header file.", w189) -> (resulting string=w190:string)  [unwired: 2 in, 1 out]
                                n60 = call "Window-Error message.vi"("Message"=w190) -> ()  [unwired: 10 in, 1 out]
                                }
                                }
                              }
                            }
                          }
                          n61 = disable-structure shown="Disabled" {
                            disable-tunnel: w151 -> [w158 w160]
                            disable-tunnel: w150 -> [w157 w159]
                            disable-tunnel: [w156 w160] -> w149
                            disable-tunnel: [w155 w159] -> w148
                            disable-tunnel: w146 -> [w154 _]
                            disable-tunnel: w145 -> [w153 _]
                            frame Disabled {
                              n62 = call "Experiment header-Maintenance.vi"("error in (no error)"=w157, "<Valid parameter names>"=w154, "section"=w153, "Experiment header file ref in"=w158) -> ("error out"=w155:errorcluster, "Experiment header file ref"=w156:T30)  [unwired: 6 in]
                            }
                            frame Enabled {
                            }
                          }
                        }
                        frame True {
                          w221 = "*.dat"  # pattern
                          # "Gets the number of trials\nin the case of Rig 2 data format."
                          # "File does not exist so it is created. HANDLES RIG 2 DATA FORMAT ONLY."
                          n63 = Array Size(array=w216) -> (size(s)=w219:i32)
                          n64 = Initialize Array(0.0, w219) -> (w203:dbl[])
                          n65 = Build Path(base path=w215, name or relative path="Points_data") -> (appended path=w220:path)
                          n66 = To Lower Case(string="Number of Trials" ("element")) -> (all lower case string=w213:string)
                          n67 = Concatenate Strings("*_PMC_G0_ChA_" ("string"), w221) -> (w222:string)
                          n68 = Search 1D Array(1D array=w212, element=w213) -> (index of element=w210:i32)  [unwired: 1 in]
                          n69 = call <vilib>:"Recursive File List.vi"("pattern"=w222, "Folder Path"=w220) -> ("error out"=w201:errorcluster, "Number of Files"=w208:i32)  [unwired: 5 in, 3 out]
                          n70 = To Double Precision Float(number=w208) -> (double precision float=w217:dbl)
                          n71 = Not Equal To 0?(x=w208) -> (x != 0?=w207:bool)
                          n72 = Not Equal?(x=w210, y=-1) -> (x != y?=w206:bool)
                          n73 = Insert Into Array(array=w203, index=w210, new element=w217) -> (w204:dbl[])
                          n74 = Compound Arithmetic op=AND(invert w201, w207, w206) -> (w205:bool)
                          n75 = Select(t=w204, s=w205, f=w203) -> (s? t:f=w202:dbl[])
                          n76 = for {
                            shift-right: [w236] -> w226
                            shift-left: w228 -> [w237]
                            tunnel: w227 -> [w235]
                            tunnel: [w234] -> w225
                            tunnel: w216 -> [w231] mode=indexing
                            tunnel: w202 -> [w229] mode=indexing
                            tunnel: w212 -> [w232]
                            tunnel: w211 -> [w230]
                            n77 = Search 1D Array(1D array=w232, element=w231) -> (index of element=w233:i32)  [unwired: 1 in]
                            n78 = call-poly <vilib>:"Write Key.vi"("section"=w235, "value"=w229, "key"=w231, "refnum"=w237) -> ("error out"=w234:errorcluster, "refnum out"=w236:T30)  [unwired: 5 in, 1 out]
                            n79 = case shown="Default" w233 {
                              selector: w233 -> [_ w245]
                              tunnel: w231 -> [w238 w242]
                              tunnel: w230 -> [_ w244]
                              tunnel: w229 -> [_ w241]
                              frame -1 {
                                # "Not found in the \"All parameters\" typedef cluster"
                                n80 = Format Into String(format string="Development error when loading header file.\nThe header parameter \"%s\" does not exist in the \"All header parameters\" enum. Add it or ensure parameter names match among all header specifier typedef clusters.", w238) -> (resulting string=w239:string)  [unwired: 2 in, 1 out]
                                n81 = call "Window-Error message.vi"("Message"=w239) -> ()  [unwired: 10 in, 1 out]
                              }
                              frame Default {
                                # "Found in the \"All parameters\" typedef cluster"
                                n82 = Index Array(array=w244, index=w245) -> (element=w246:refnum<vi>)
                                n83 = property class="Ctl"(reference=w246, "Value"=w241) -> (error out=w243:errorcluster)  [unwired: 1 in, 1 out]
                                n84 = case shown="Error" w243 {
                                tunnel: w242 -> [_ w248]
                                frame No Error {
                                }
                                frame Error {
                                n85 = Format Into String(format string="The header parameter \"%s\" cannot be handled. The code may need to be upgraded to allow reading non-numeric parameter values from the header file.", w248) -> (resulting string=w249:string)  [unwired: 2 in, 1 out]
                                n86 = call "Window-Error message.vi"("Message"=w249) -> ()  [unwired: 10 in, 1 out]
                                }
                                }
                              }
                            }
                          }
                        }
                      }
                    }
                    frame "Save file" {
                      # "Filters in only the parameters which exist in the selected data structure depending on the data header type."
                      n87 = call "Experiment header-Write LOGIN section.vi"("error in (no error)"=w254, "Experiment header file ref"=w264) -> ("error out"=w251:errorcluster, "Experiment header file ref"=w255:T30)  [unwired: 8 in]
                      n88 = call "Experiment header-Gen user name stamp file.vi"("error in (no error)"=w251, "Experiment data folder path"=w252) -> ("error out"=w250:errorcluster)  [unwired: 9 in]
                      n89 = property on="All header parameters in" class="Clust (strict)"(error in=w250) -> (error out=w253:errorcluster, "Controls[]"=w262:refnum<vi>[])  [unwired: 1 in, 1 out]
                      n90 = for {
                        shift-right: [w274] -> w261
                        shift-left: w255 -> [w275]
                        tunnel: w266 -> [w273]
                        tunnel: w265 -> [w270] mode=indexing
                        tunnel: w263 -> [w271]
                        tunnel: w262 -> [w269]
                        tunnel: [w268] -> w259
                        tunnel: w253 -> [w267]
                        # "...find its index in the global parameters cluster"
                        # "FOR each parameter in the current header type..."
                        n91 = Search 1D Array(1D array=w271, element=w270) -> (index of element=w272:i32)  [unwired: 1 in]
                        n92 = case shown="Default" w272 {
                          selector: w272 -> [_ w291]
                          tunnel: w275 -> [w279 w294]
                          tunnel: [w279 w293] -> w274
                          tunnel: w273 -> [_ w292]
                          tunnel: w270 -> [w278 w283]
                          tunnel: w269 -> [_ w287]
                          tunnel: [_ w281] -> w268
                          tunnel: w267 -> [_ w280]
                          frame -1 {
                            # "Not found in the \"All parameters\" typedef cluster"
                            n93 = Format Into String(format string="Development error when writing header file.\nThe header parameter \"%s\" does not exist in the \"All header parameters\" enum. Add it or ensure parameter names match among all header specifier typedef clusters.", w278) -> (resulting string=w277:string)  [unwired: 2 in, 1 out]
                            n94 = call "Window-Error message.vi"("Message"=w277) -> ()  [unwired: 10 in, 1 out]
                          }
                          frame Default {
                            # "Warning!\nCannot handle paths or other control types \nwhose value cannot be converter to a number."
                            # "Found in the \"All parameters\" typedef cluster"
                            n95 = Index Array(array=w287, index=w291) -> (element=w290:refnum<vi>)
                            n96 = property class="Ctl"(reference=w290, error in=w280) -> (error out=w285:errorcluster, "Value"=w289:variant)  [unwired: 1 out]
                            n97 = Variant To Data(error in=w285, type=0.0, Variant=w289) -> (data=w286:dbl, error out=w284:errorcluster)
                            n98 = call-poly <vilib>:"Write Key.vi"("section"=w292, "error in (no error)"=w284, "value"=w286, "key"=w283, "refnum"=w294) -> ("error out"=w282:errorcluster, "refnum out"=w293:T30)  [unwired: 4 in, 1 out]
                            n99 = case shown="Error" w284 {
                              tunnel: w283 -> [_ w295]
                              frame No Error {
                              }
                              frame Error {
                                n100 = Format Into String(format string="The header parameter \"%s\" cannot be handled. The code may need to be upgraded to allow write/read non-numeric parameter values to the header file.", w295) -> (resulting string=w296:string)  [unwired: 2 in, 1 out]
                                n101 = call "Window-Error message.vi"("Message"=w296) -> ()  [unwired: 10 in, 1 out]
                              }
                            }
                            n102 = call <vilib>:"Clear Errors.vi"("error in (no error)"=w282) -> ("error out"=w281:errorcluster)  [unwired: 5 in, 1 out]
                          }
                        }
                      }
                      n103 = call "Experiment header-Save_Load mov cor section.vi"("Input Mode (ref)"=enum16{"Use reference", "Use folder path"}."Use reference", "error in (no error)"=w259, "Function"=enum16{"Write", "Read"}."Write", "Exp header file ref in"=w261) -> ("error out"=w260:errorcluster, "Exp header file ref"=w258:T30)  [unwired: 5 in, 1 out]
                    }
                  }
                  n104 = call <vilib>:"Close Config Data.vi"("error in (no error)"=w129, "refnum"=w130) -> ("error out"=w128:errorcluster)  [unwired: 8 in, 1 out]
                }
                frame Error {
                }
              }
              n105 = case shown="Error" w112 {
                selector: w112 -> [_ w310]
                tunnel: [_ w310] -> w101
                tunnel: w105 -> [w301 _]
                tunnel: w99 -> [w300 _]
                tunnel: w110 -> [w299 _]
                frame No Error {
                  n106 = disable-structure shown="Disabled" {
                    disable-tunnel: w301 -> [w304 _]
                    disable-tunnel: w300 -> [w303 _]
                    disable-tunnel: w299 -> [w302 _]
                    frame Disabled {
                      n107 = case shown="True" w304 {
                        tunnel: w303 -> [_ w307]
                        tunnel: w302 -> [_ w305]
                        frame False {
                        }
                        frame True {
                          n108 = Path To String(path=w307) -> (string=w306:string)
                          n109 = Format Into String(format string="\"%s\" file was created in:\n\n%s" ("message"), w305, w306) -> (resulting string=w308:string)  [unwired: 2 in, 1 out]
                          n110 = One Button Dialog(message=w308) -> ()  [unwired: 1 in, 1 out]
                        }
                      }
                    }
                    frame Enabled {
                    }
                  }
                }
                frame Error {
                }
              }
              n111 = case shown="\"Save file\", \"Save file as\"" w100 {
                tunnel: [w116 w119] -> w102
                tunnel: w101 -> [w116 w118]
                tunnel: w99 -> [_ w117]
                frame Default {
                }
                frame "Save file", "Save file as" {
                  n112 = call "Exp header-Save cal header info.vi"("error in (no error)"=w118, "Experiment folder path"=w117) -> ("error out"=w119:errorcluster)  [unwired: 9 in]
                }
              }
            }
            frame True {
              # "Folder foes not exist! OR Error"
              n113 = case shown="No Error" w311 {
                selector: w311 -> [_ w322]
                tunnel: w313 -> [w319 _]
                tunnel: [w317 w322] -> w312
                frame No Error {
                  n114 = Path To String(path=w319) -> (string=w320:string)
                  n115 = Format Into String(format string="\"Experiment Header.ini\" file could not be accessed because the specified folder path does not exist.\n\nPath:\n%s" ("message"), w320) -> (resulting string=w314:string)  [unwired: 2 in, 1 out]
                  n116 = call "Window-Error message.vi"("Message"=w314) -> ()  [unwired: 10 in, 1 out]
                  n117 = Bundle By Name(cluster=errorcluster {"status"=FALSE, "code"=0, "source"=""} ("error out"), "source"=w314, "status"=TRUE, "code"=5000) -> (w317:errorcluster)
                }
                frame Error {
                }
              }
            }
          }
        }
      }
    }
    frame Enabled {
    }
  }
  n118 = flat-sequence {
    tunnel: w2 -> [w323]
    tunnel: [w323] -> w1
    frame #0 {
    }
  }
  "error out" <- w1
